vi "ejercicio 9.vi"(4 "Número C":dbl, 5 "Número A":dbl, 6 "Número B":dbl) -> (0 "Discriminante < 0":bool, 1 "Discriminante = 0":bool, 2 "Discriminante > 0":bool, 3 "Discriminante":dbl)   [LabVIEW 2015]
doc: "Este VI representa el discriminante de un número.\nCada diodo se enciende de acuerdo al valor del discriminante."
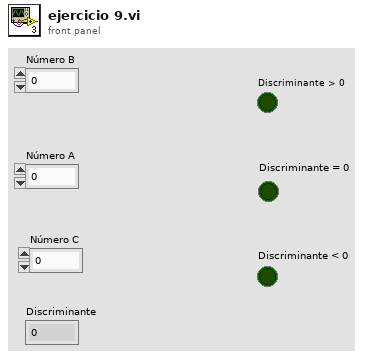
[diagram p1: front panel]
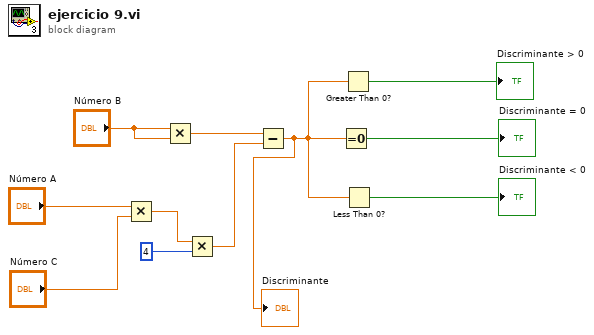
[diagram p0: block diagram]
diagram:
  n1 = Multiply(x="Número A", y="Número C") -> (x*y=w2:dbl)
  n2 = Multiply(x="Número B", y="Número B") -> (x*y=w10:dbl)
  n3 = Multiply(x=w2, y=4) -> (x*y=w1:dbl)
  n4 = Subtract(x=w10, y=w1) -> (x-y=w4:dbl)
  "Discriminante" <- w4
  n5 = Equal To 0?(x=w4) -> (x = 0?=→"Discriminante = 0":bool)
  n6 = Greater Than 0?(x=w4) -> (x > 0?=→"Discriminante > 0":bool)
  n7 = Less Than 0?(x=w4) -> (x < 0?=→"Discriminante < 0":bool)
